vi "Init.vi"(8 "error in (no error)":errorcluster, 11 "Report Generator In":refnum<class "Report Generator.lvclass">) -> (0 "error out":errorcluster, 3 "Report Generator Out":refnum<class "Report Generator.lvclass">)   [LabVIEW 2020, in "Reports.lvlib" / "Report Generator.lvclass"]
uses:
  Report Generator.lvclass
  User Interface/Process/Process.lvclass
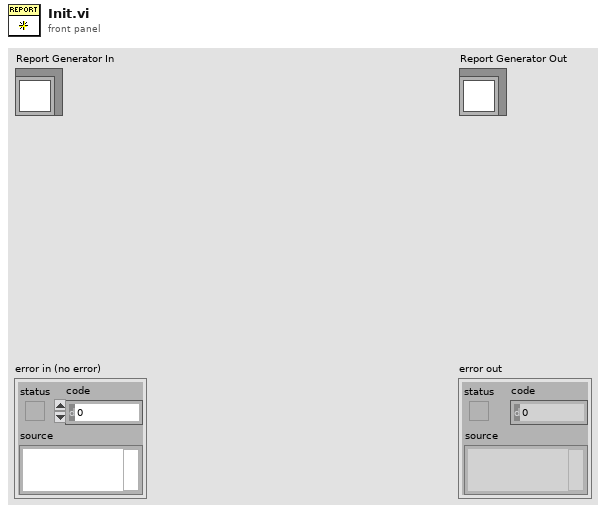
[diagram p1: front panel]
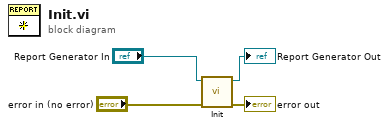
[diagram p0: block diagram]
diagram:
  n1 = call-parent "Init.vi"("error in (no error)"="error in (no error)", "Process In"="Report Generator In") -> ("error out"=→"error out":errorcluster, "Process Out"=→"Report Generator Out":refnum<class "Report Generator.lvclass">)  [unwired: 8 in]
